vi "GlobalLabVIEWStart.vi"() -> ()   [LabVIEW 2015]
panel:
  in  "LabVIEW Speed Channels":dbl[](array[numeric])
  in  "LabVIEW Start":dbl
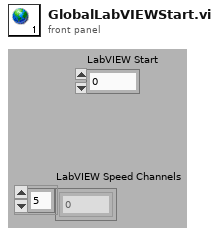
[diagram p1: front panel]
diagram:
